vi "Func Processor for K-Laws.vi"(8 "Math Expressions In":string[](array[string]), 9 "Fn Arg Cnt":string[](array[string]), 10 "Functions Definition":string[][](table), 11 "Total Function Definitions":i32) -> (3 "Math Expressions Out":string[](array[string]))   [LabVIEW 2014]
panel:
  out "Function Formula":string
  out "Fn-Math":string[](array[string])
  out "Fn Name":string[](array[string])
  # "External Inputs"
  # "Intermediate variables"
  # "Outputs"
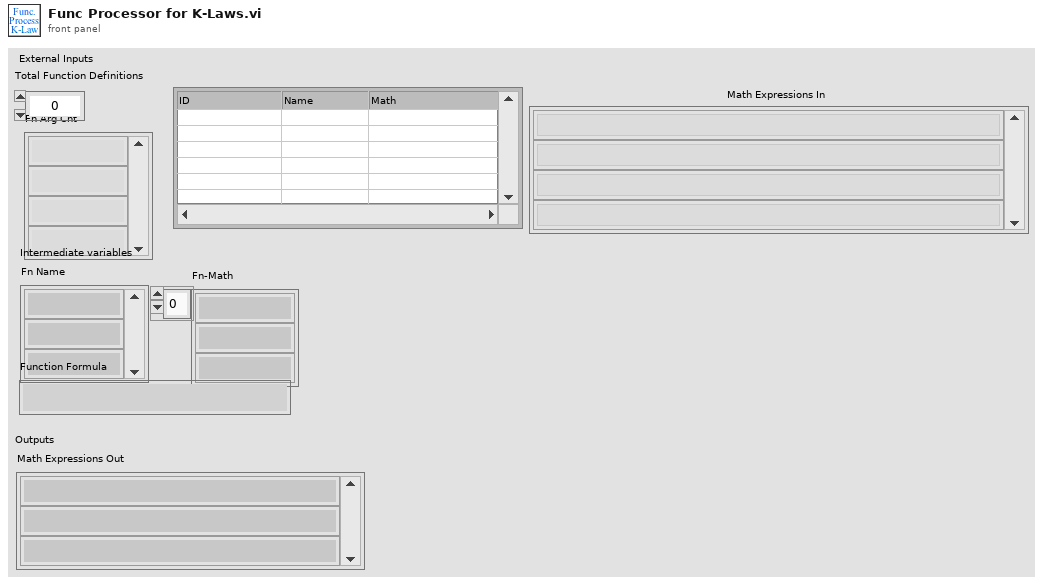
[diagram p1: front panel]
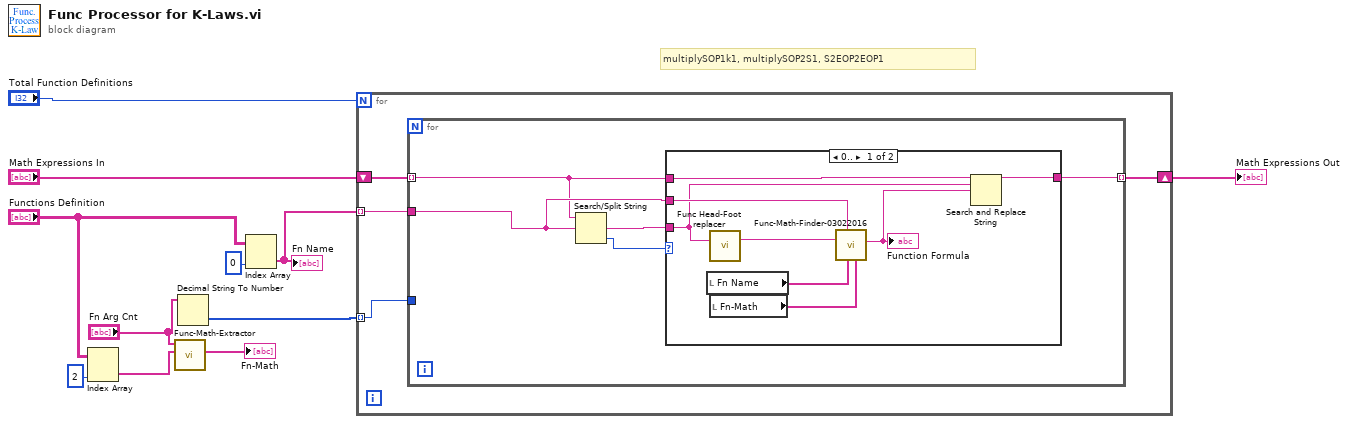
[diagram p0: block diagram]
diagram:
  # "multiplySOP1k1, multiplySOP2S1, S2EOP2EOP1"
  n1 = Index Array(array="Functions Definition", index (col)=2 ("disabled index (col)")) -> (element=w5:string[])  [unwired: 1 in]
  n2 = call "Func-Math-Extractor.vi"("Fn Math"=w5, "Fn Arg Cnt"="Fn Arg Cnt") -> ("Fn-Math"=→"Fn-Math":string[])  [unwired: 9 in]
  n3 = Decimal String To Number(string="Fn Arg Cnt") -> (number=w3:i32[])  [unwired: 2 in, 1 out]
  n4 = Index Array(array="Functions Definition", index (col)=0 ("disabled index (col)")) -> (element=w7:string[])  [unwired: 1 in]
  "Fn Name" <- w7
  n5 = for {
    N: "Total Function Definitions" -> [_]
    tunnel: w7 -> [w14] mode=indexing
    tunnel: w3 -> [w13] mode=indexing
    shift-right: [w12] -> w1
    shift-left: "Math Expressions In" -> [w15]
    n6 = for {
      tunnel: w15 -> [w17] mode=indexing
      tunnel: w14 -> [w19]
      tunnel: w13 -> [_]
      tunnel: [w16] -> w12 mode=indexing
      n7 = Search/Split String(string=w17, search string/char (-)=w19) -> (match + rest of string=w20:string, offset of match=w18:i32)  [unwired: 1 in, 1 out]
      n8 = case shown="0.." w18 {
        tunnel: w20 -> [w23 _]
        tunnel: w19 -> [w27 _]
        tunnel: w17 -> [w24 w29]
        tunnel: [w21 w29] -> w16
        frame 0.. {
          n9 = local read "Fn Name"() -> (w26:string[])
          n10 = call "Func Head-Foot replacer.vi"("Function in"=w23) -> ("Function in Out"=w28:string)  [unwired: 12 in, 2 out]
          n11 = local read "Fn-Math"() -> (w25:string[])
          n12 = call "Func-Math-Finder-03022016.vi"("All Fn-Math"=w25, "All Fn Name"=w26, "Func Name"=w27, "Get Tagged String"=w28) -> ("Expression"=w22:string)  [unwired: 5 in, 2 out]
          "Function Formula" <- w22
          n13 = Search and Replace String(input string=w24, search string=w23, replace string=w22) -> (result string=w21:string)  [unwired: 5 in, 3 out]
        }
        frame -1, Default {
        }
      }
    }
  }
  "Math Expressions Out" <- w1
